vi "Set SET parameters.vi"(8 "error in (no error)":errorcluster, 11 "CCDCamera in":refnum<class "CCDCamera.lvclass">) -> (0 "error out":errorcluster, 2 "new parameter":bool, 3 "CCDCamera out":refnum<class "CCDCamera.lvclass">)   [LabVIEW 2018, in "CCDCamera.lvclass"]
uses:
  CCDCamera.lvclass
  Simulated_CCD_Camera/Simulated_CCD_Camera.lvclass
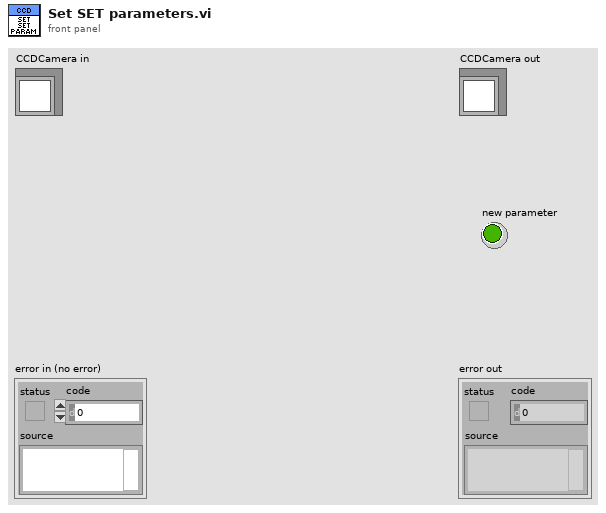
[diagram p1: front panel]
types:
  T1 = cluster{"COOLER_POWER_STATUS":u16, "TEMP":i32, "EXPTIME":sgl, "#FRAMES":u32, "#CUBES":u32}
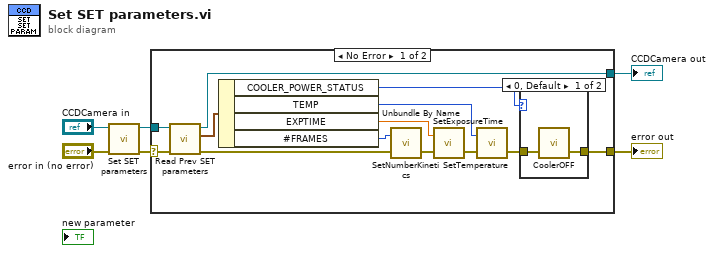
[diagram p0: block diagram]
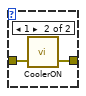
[diagram p2: hidden frame]
diagram:
  n1 = call-parent "Set SET parameters.vi"("error in (no error)"="error in (no error)", "Simulated_CCD_Camera in"="CCDCamera in") -> ("error out"=w4:errorcluster, "Simulated_CCD_Camera out"=w3:refnum<class "CCDCamera.lvclass">)  [unwired: 7 in, 1 out]
  n2 = case shown="No Error" w4 {
    selector: w4 -> [w19 w24]
    tunnel: w3 -> [w18 w25]
    tunnel: [w8 w24] -> w2
    tunnel: [w7 w25] -> w1
    frame No Error {
      n3 = call-dynamic "Read Prev SET parameters.vi"("error in (no error)"=w19, "Simulated_CCD_Camera in"=w18) -> ("error out"=w12:errorcluster, "Prev SET parameters"=w17:T1, "Simulated_CCD_Camera out"=w7:refnum<class "CCDCamera.lvclass">)  [unwired: 7 in]
      n4 = Unbundle By Name(w17) -> ("COOLER_POWER_STATUS"=w13:u16, "TEMP"=w14:i32, "EXPTIME"=w15:sgl, "#FRAMES"=w16:u32)
      n5 = call <userlib>:"SetNumberKinetics.vi"("error in (no error)"=w12, "number"=w16) -> ("error out"=w11:errorcluster)  [unwired: 1 out]
      n6 = call <userlib>:"SetExposureTime.vi"("error in (no error)"=w11, "time"=w15) -> ("error out"=w10:errorcluster)  [unwired: 1 out]
      n7 = call <userlib>:"SetTemperature.vi"("error in (no error)"=w10, "temperature"=w14) -> ("error out"=w9:errorcluster)  [unwired: 1 out]
      n8 = case shown="0, Default" w13 {
        tunnel: w9 -> [w21 w23]
        tunnel: [w20 w22] -> w8
        frame 0, Default {
          n9 = call <userlib>:"CoolerOFF.vi"("error in (no error)"=w21) -> ("error out"=w20:errorcluster)  [unwired: 1 in, 1 out]
        }
        frame 1 {
          n10 = call <userlib>:"CoolerON.vi"("error in (no error)"=w23) -> ("error out"=w22:errorcluster)  [unwired: 1 in, 1 out]
        }
      }
    }
    frame Error {
    }
  }
  "error out" <- w2
  "CCDCamera out" <- w1
